vi "SEED TABLES.vi"(8 "error in":errorcluster, 11 "LV-ORM in":refnum<class "LV-ORM.lvclass">) -> (0 "error out":errorcluster, 3 "LV-ORM out":refnum<class "LV-ORM.lvclass">)   [LabVIEW 2018, in "LV-ORM.lvclass"]
uses:
  LV-ORM.lvclass
  demo/Implementations/Component-A.lvclass
  demo/Implementations/Product-A.lvclass
  U:/modules/labview-orm/_Serializable Base Object/_ISerializable.lvclass
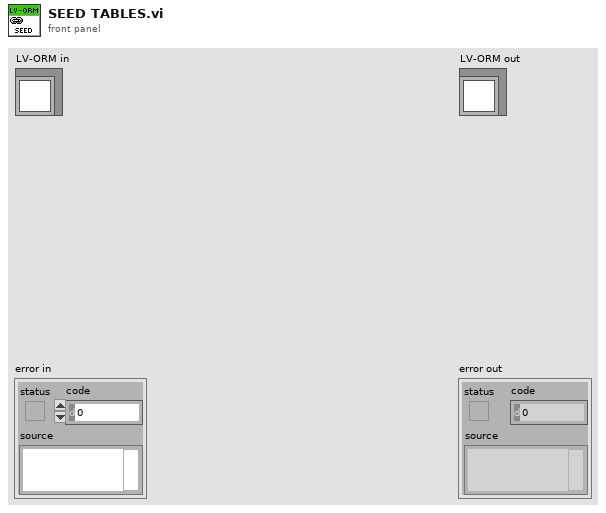
[diagram p1: front panel]
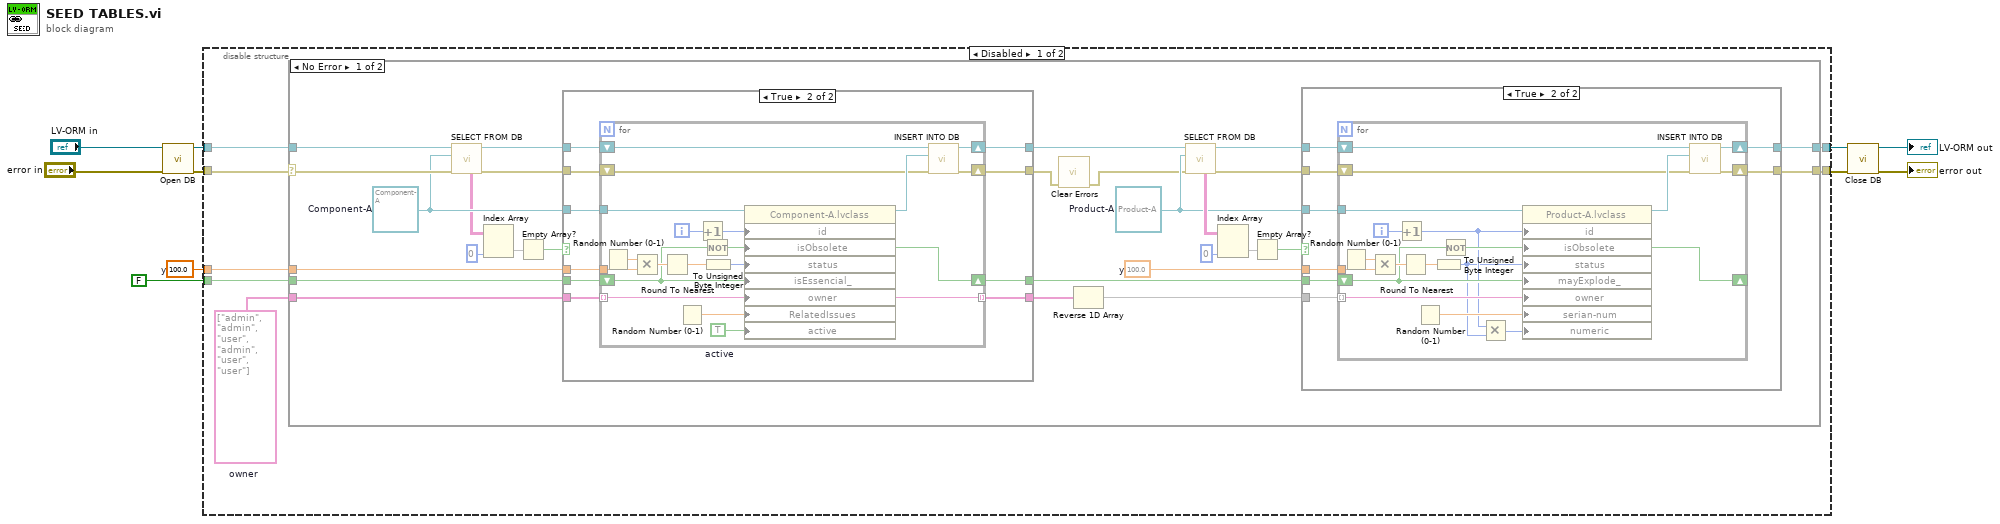
[diagram p0: block diagram]
diagram:
  w2 = 100.0  # y
  n1 = call "Open DB.vi"("error in (no error)"="error in", "LV-ORM in"="LV-ORM in") -> ("error out"=w7:errorcluster, "LV-ORM out"=w9:refnum<class "LV-ORM.lvclass">)  [unwired: 8 in]
  n2 = disable-structure shown="Disabled" {
    disable-tunnel: w9 -> [w17 w109]
    disable-tunnel: w7 -> [w16 w108]
    disable-tunnel: [w15 w109] -> w6
    disable-tunnel: [w14 w108] -> w5
    disable-tunnel: w2 -> [w12 _]
    disable-tunnel: FALSE -> [w11 _]
    frame Disabled {
      w13 = string[] ["admin", "admin", "user", "admin", "user", "user"]  # owner
      n3 = case shown="No Error" w16 {
        selector: w16 -> [w36 w107]
        tunnel: [w41 w107] -> w14
        tunnel: [w42 w106] -> w15
        tunnel: w17 -> [w37 w106]
        tunnel: w13 -> [w45 _]
        tunnel: w12 -> [w44 _]
        tunnel: w11 -> [w43 _]
        frame No Error {
          w39 = 100.0  # y
          w35 = refnum<class "Component-A.lvclass"> refnum  # Component-A
          w25 = refnum<class "Product-A.lvclass"> refnum  # Product-A
          n4 = call "SELECT FROM DB.vi"("error in"=w36, "object"=w35, "orm in"=w37) -> ("error out"=w29:errorcluster, "orm out"=w30:refnum<class "LV-ORM.lvclass">, "data"=w34:string[][])  [unwired: 4 in, 2 out]
          n5 = Index Array(array=w34, index (col)=0) -> (element=w32:string[])  [unwired: 1 in]
          n6 = Empty Array?(array=w32) -> (empty?=w31:bool)
          n7 = case shown="True" w31 {
            tunnel: w30 -> [w77 w87]
            tunnel: w29 -> [w76 w86]
            tunnel: w45 -> [w74 w85]
            tunnel: w44 -> [_ w84]
            tunnel: w43 -> [w75 w83]
            tunnel: [w77 w82] -> w23
            tunnel: w35 -> [_ w81]
            tunnel: [w75 w80] -> w40
            tunnel: [w74 w79] -> w19
            tunnel: [w76 w78] -> w38
            frame False {
            }
            frame True {
              n8 = for {
                tunnel: w81 -> [w105]
                shift-right: [w104] -> w82
                shift-left: w87 -> [w103]
                shift-right: [w100] -> w78
                shift-left: w86 -> [w101]
                tunnel: w85 -> [w89] mode=indexing
                tunnel: w84 -> [w92]
                shift-right: [w90] -> w80
                shift-left: w83 -> [w91]
                tunnel: [w89] -> w79 mode=indexing
                i -> [w98]
                w88 = TRUE  # active
                n9 = Random Number (0-1)() -> (number: 0 to 1=w96:dbl)
                n10 = Multiply(x=w96, y=w92) -> (x*y=w95:dbl)
                n11 = Round To Nearest(number=w95) -> (nearest integer value=w94:dbl)
                n12 = Random Number (0-1)() -> (number: 0 to 1=w99:dbl)
                n13 = Increment(x=w98) -> (x+1=w97:i32)
                n14 = Not(x=w91) -> (.not. x?=w90:bool)
                n15 = To Unsigned Byte Integer(number=w94) -> (unsigned 8bit integer=w93:u8)
                n16 = property class="Component-A.lvclass"(reference=w105, "id"=w97, "isObsolete"=w90, "status"=w93, "isEssencial_"=w91, "owner"=w89, "RelatedIssues"=w99, "active"=w88) -> (reference out=w102:refnum<class "Component-A.lvclass">)  [unwired: 1 in, 1 out]
                n17 = call "INSERT INTO DB.vi"("error in"=w101, "object"=w102, "orm in"=w103) -> ("error out"=w100:errorcluster, "orm out"=w104:refnum<class "LV-ORM.lvclass">)  [unwired: 7 in]
              }
            }
          }
          n18 = call <vilib>:"Clear Errors.vi"("error in (no error)"=w38) -> ("error out"=w22:errorcluster)  [unwired: 5 in, 1 out]
          n19 = Reverse 1D Array(array=w19) -> (reversed array=w18:string[])
          n20 = call "SELECT FROM DB.vi"("error in"=w22, "object"=w25, "orm in"=w23) -> ("error out"=w21:errorcluster, "orm out"=w20:refnum<class "LV-ORM.lvclass">, "data"=w26:string[][])  [unwired: 4 in, 2 out]
          n21 = Index Array(array=w26, index (col)=0) -> (element=w28:string[])  [unwired: 1 in]
          n22 = Empty Array?(array=w28) -> (empty?=w24:bool)
          n23 = case shown="True" w24 {
            tunnel: [w47 w55] -> w42
            tunnel: [w46 w54] -> w41
            tunnel: w25 -> [_ w53]
            tunnel: w40 -> [_ w52]
            tunnel: w18 -> [_ w51]
            tunnel: w39 -> [_ w50]
            tunnel: w21 -> [w46 w49]
            tunnel: w20 -> [w47 w48]
            frame False {
            }
            frame True {
              n24 = for {
                tunnel: w53 -> [w73]
                shift-right: [w72] -> w55
                shift-left: w48 -> [w71]
                shift-right: [w68] -> w54
                shift-left: w49 -> [w69]
                tunnel: w51 -> [w65] mode=indexing
                tunnel: w50 -> [w61]
                shift-right: [w59] -> _
                shift-left: w52 -> [w60]
                i -> [w66]
                n25 = Random Number (0-1)() -> (number: 0 to 1=w64:dbl)
                n26 = Multiply(x=w64, y=w61) -> (x*y=w63:dbl)
                n27 = Increment(x=w66) -> (x+1=w58:i32)
                n28 = Round To Nearest(number=w63) -> (nearest integer value=w62:dbl)
                n29 = Random Number (0-1)() -> (number: 0 to 1=w67:dbl)
                n30 = To Unsigned Byte Integer(number=w62) -> (unsigned 8bit integer=w57:u8)
                n31 = Not(x=w60) -> (.not. x?=w59:bool)
                n32 = Multiply(x=w58, y=w57) -> (x*y=w56:i32)
                n33 = property class="Product-A.lvclass"(reference=w73, "id"=w58, "isObsolete"=w59, "status"=w57, "mayExplode_"=w60, "owner"=w65, "serian-num"=w67, "numeric"=w56) -> (reference out=w70:refnum<class "Product-A.lvclass">)  [unwired: 1 in, 1 out]
                n34 = call "INSERT INTO DB.vi"("error in"=w69, "object"=w70, "orm in"=w71) -> ("error out"=w68:errorcluster, "orm out"=w72:refnum<class "LV-ORM.lvclass">)  [unwired: 7 in]
              }
            }
          }
        }
        frame Error {
        }
      }
    }
    frame Enabled {
    }
  }
  n35 = call "Close DB.vi"("error in"=w5, "LV-ORM in"=w6) -> ("error out"=→"error out":errorcluster, "LV-ORM out"=→"LV-ORM out":refnum<class "LV-ORM.lvclass">)  [unwired: 8 in]
